vi "Add new entry.vi"(8 "error in (no error)":errorcluster, 9 "Severity":string="error", 10 "Text to log":string, 11 "SysLogbook in":refnum<class "SysLogbook.lvclass">) -> (0 "error out":errorcluster, 3 "SysLogbook out":refnum<class "SysLogbook.lvclass">)   [LabVIEW 2014, in "SysLogbook.lvclass"]
doc: "Sends a msg to syslog collector\n\nSeverity: emergency; alert; critical; error; warning; notice; info"
uses:
  SysLogbook.lvclass
  <vilib>/NI/syslog/_subVIs/TypeDefs/syslog_severity_codes.ctl
  SysLogbook.lvclass/SysLogbook.ctl
  Logbook/Logbook.lvclass
panel:
  out "Syslog Message for debug":string
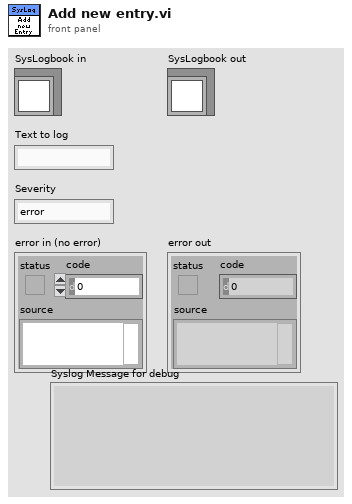
[diagram p1: front panel]
types:
  T1 = typedef "syslog_severity_codes.ctl" = enum16{"emergency", "alert", "critical", "error", "warning", "notice", "info", "debug"}
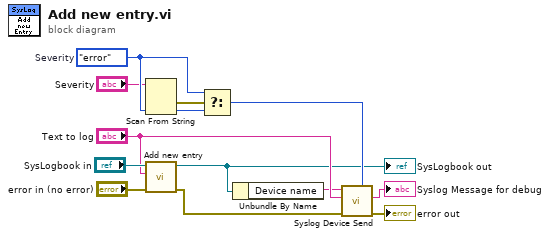
[diagram p0: block diagram]
diagram:
  w8 = syslog_severity_codes."error"  # Severity
  n1 = Scan From String(input string="Severity", default 1=w8) -> (error out=w9:errorcluster, output 1=w7:T1)  [unwired: 3 in, 2 out]
  n2 = call-parent "Add new entry.vi"("error in (no error)"="error in (no error)", "Text to log"="Text to log", "Logbook in"="SysLogbook in") -> ("error out"=w11:errorcluster, "Logbook out"=w4:refnum<class "SysLogbook.lvclass">)  [unwired: 7 in]
  "SysLogbook out" <- w4
  n3 = Select(t=w8, s=w9, f=w7) -> (s? t:f=w6:T1)
  n4 = Unbundle By Name(w4) -> ("Device name"=w3:string)
  n5 = call <vilib>:"Syslog Device Send.vi"("Severity Code (error)"=w6, "error in (no error)"=w11, "Message Content"="Text to log", "Message Tag"=w3) -> ("error out"=→"error out":errorcluster, "Syslog Message"=→"Syslog Message for debug":string)  [unwired: 6 in]
